vi "Write NetImpParams.vi"(8 "error in (no error)":errorcluster, 10 "dblNetImpParams":dbl[][](array[numeric]), 11 "NetworkImpairmentPluginBase in":refnum<class "NetworkImpairmentPluginBase.lvclass">) -> (0 "error out":errorcluster, 3 "NetworkImpairmentPluginBase out":refnum<class "NetworkImpairmentPluginBase.lvclass">)   [LabVIEW 2017, in "NetworkImpairmentPlugins.lvlib" / "NetworkImpairmentPluginBase.lvclass"]
uses:
  NetworkImpairmentPluginBase.lvclass
  NetworkImpairmentPluginBase.lvclass/NetworkImpairmentPluginBase.ctl
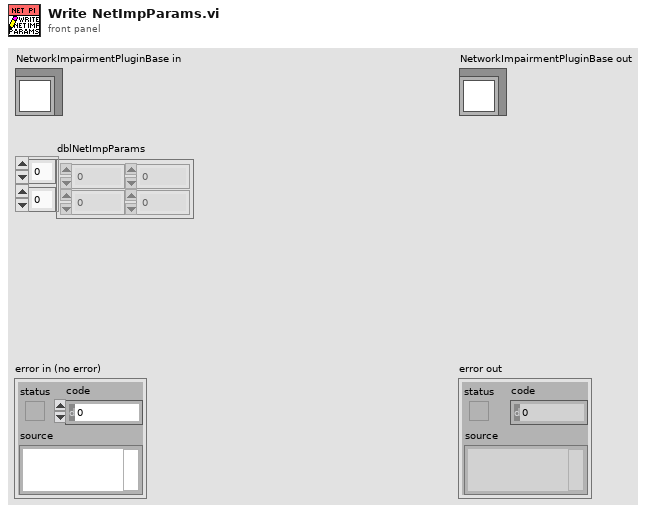
[diagram p1: front panel]
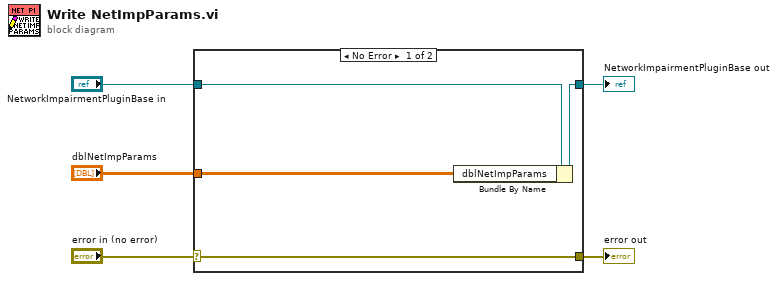
[diagram p0: block diagram]
diagram:
  n1 = case shown="No Error" "error in (no error)" {
    selector: "error in (no error)" -> [w9 w10]
    tunnel: [w9 w10] -> w4
    tunnel: [w7 w11] -> w2
    tunnel: "NetworkImpairmentPluginBase in" -> [w8 w11]
    tunnel: "dblNetImpParams" -> [w6 _]
    frame No Error {
      n2 = Bundle By Name(cluster=w8, "dblNetImpParams"=w6) -> (w7:refnum<class "NetworkImpairmentPluginBase.lvclass">)
    }
    frame Error {
    }
  }
  "error out" <- w4
  "NetworkImpairmentPluginBase out" <- w2
